vi "Module Execution Main.vi"() -> ()   [LabVIEW 2013, in "module execution process.lvlib"]
uses:
  module execution process.lvlib
  SubVIs/queue name.ctl
  SubVIs/command commands to rtexe process.ctl
  <vilib>/NI/Module Execution Interface/Engine Runtime/Engine Runtime Interface.lvclass
  <vilib>/NI/Tag Bus Module Framework/plugin discovery singleton/class discovery singleton methods.ctl
  SubVIs/engine status data.ctl
  <vilib>/NI/Module Execution Interface/Engine Runtime/Execution States.ctl
  <vilib>/NI/AMC/Read Termination Message.vi
  <vilib>/NI/AMC/Create Single Message.vi
  <vilib>/NI/AMC/Globals.vi
  <vilib>/NI/Module Execution Interface/Engine Configuration/engine configuration.lvclass
  <vilib>/NI/Tag Bus Module Framework/module configuration/TBM module configuration.lvclass
  <vilib>/NI/Tag Bus Module Framework/runtime/TBM module execution interface.lvclass
  <vilib>/nisyscfg/nisyscfg.lvlib
  Framework Configuration Classes/platypus configuration/PLConfigurationSerializer.lvlib
  <vilib>/NI/Tag Bus Module Framework/plugin discovery singleton/class discovery singleton.lvlib
  <vilib>/NI/AMC/AMC.lvlib
panel:
  out "error out":errorcluster
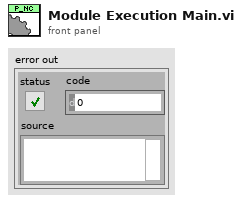
[diagram p1: front panel]
types:
  T1 = typedef "module execution process.lvlib/command commands to rtexe process.ctl" = enum16{"Initialize", "Load from File", "Load from String", "Open All Engines", "Open Single Engine", "Initialize All Engines", "Initialize Single Engine", "Start All", "Start Single", "Pause All", "Pause Single", "Stop All", "Stop Single", "Close All", "Close Single", "Set Safe State All", "Set Safe State Single", "Get Status", "Exit", "Error", "Add Search Paths"}
  T2 = typedef "module execution process.lvlib/queue name.ctl" = enum16{"TOrtmainexec", "FROMrtmainexec"}
  T3 = typedef "AMC.lvlib/Message Queue.ctl" = refnum<queue>
  T4 = typedef "class discovery singleton.lvlib/class discovery singleton methods.ctl" = enum16{"add search paths", "load class by name", "list available classes", "get class path"}
  T5 = typedef "module execution process.lvlib/engine status data.ctl" = cluster{"Name":string, "Engine State":T6, "Engine Error":errorcluster}
  T6 = typedef "Engine Runtime Interface.lvclass/Execution States.ctl" = enum16{"Initializing", "Paused (Initialized)", "Running", "Set Safe Outputs", "Uninitializing", "Stopped (Uninitialized)", "Error (Uninitialized)", "Safe State (Uninitialized)", "Closed"}
  T7 = typedef "module execution process.lvlib/configuration elements.ctl" = cluster{"Name":string, "opened?":bool, "configuration":T8, "engine":refnum<class "Engine Runtime Interface.lvclass">, "modules":refnum<class "TBM module execution interface.lvclass">[]}
  T8 = typedef "PLConfigurationSerializer.lvlib/engines cluster.ctl" = cluster{"engine configuration":refnum<class "engine configuration.lvclass">, "modules":refnum<class "TBM module configuration.lvclass">[]}
  T9 = typedef "PLConfigurationSerializer.lvlib/systems cluster.ctl" = cluster{"System Configuration":refnum<class "PL_System Configuration.lvclass">, "targets":T10[]}
  T10 = typedef "PLConfigurationSerializer.lvlib/targets cluster.ctl" = cluster{"Target Configuration":refnum<class "PL_Target Configuration.lvclass">, "engines":T8[]}
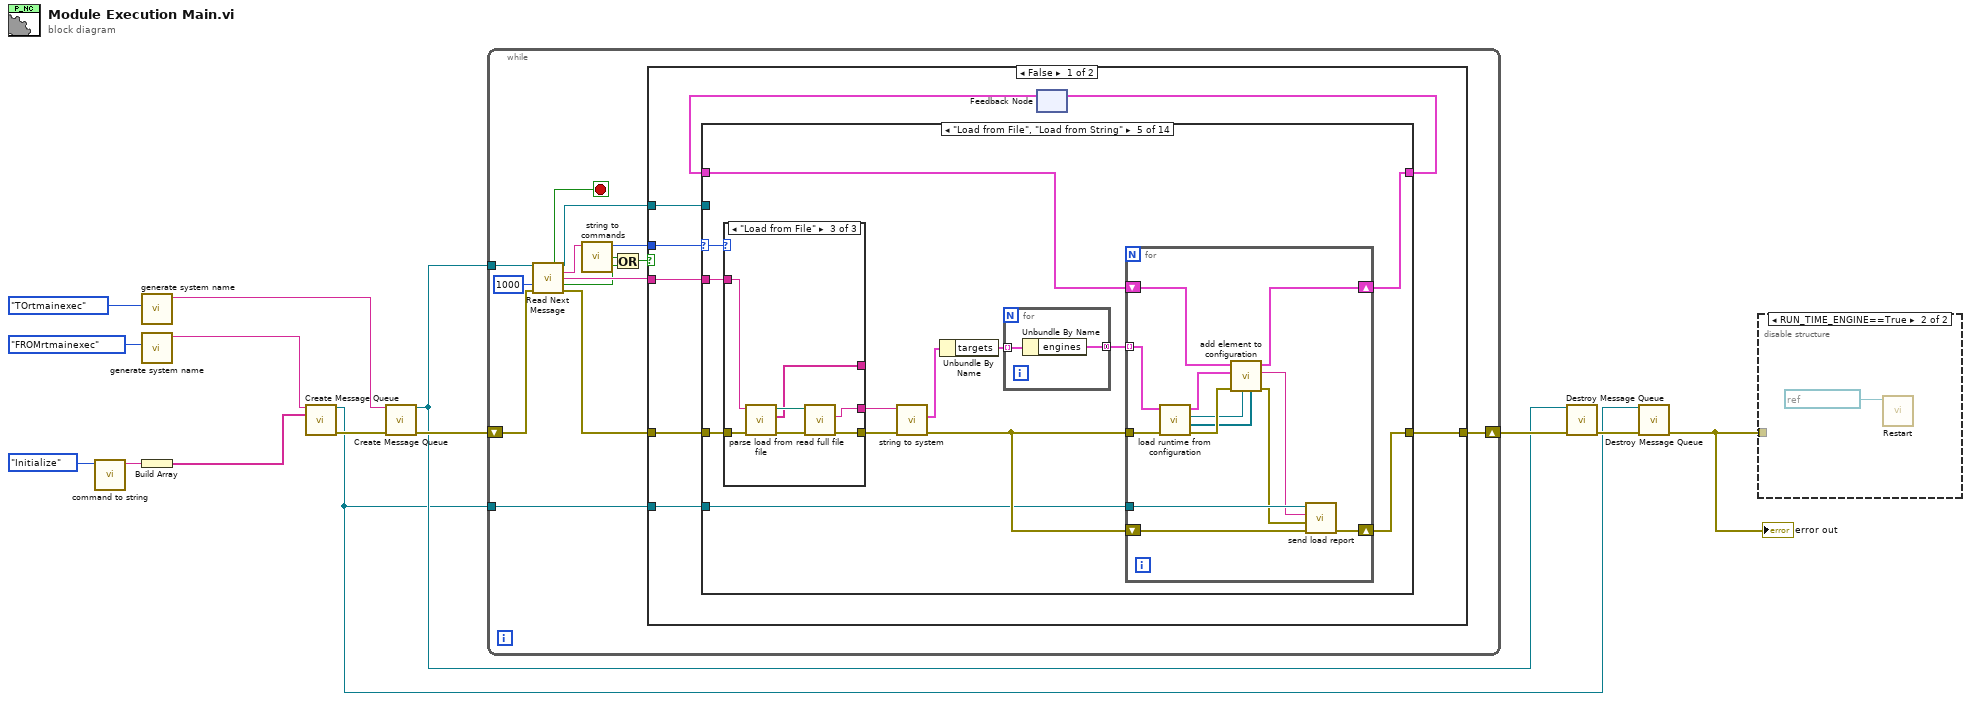
[diagram p0: block diagram]
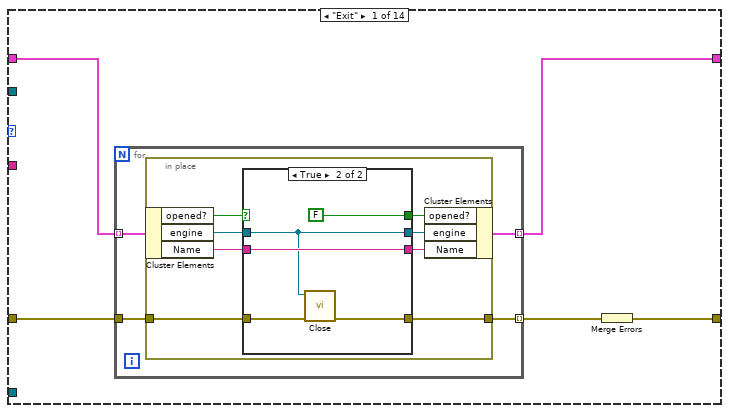
[diagram p3: hidden frame]
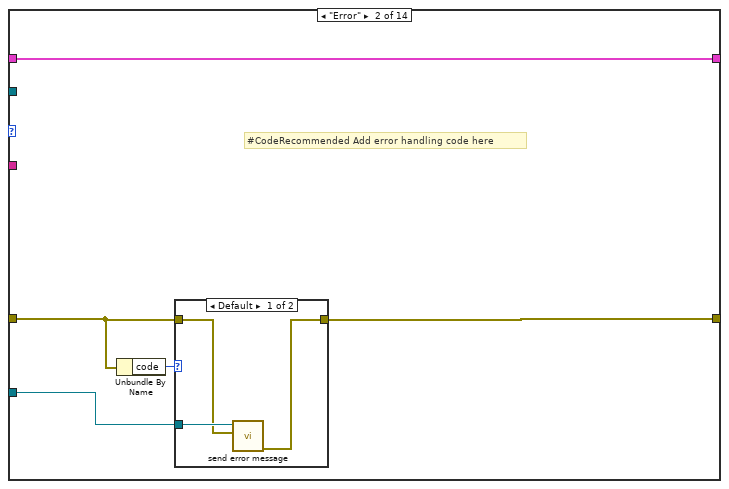
[diagram p5: hidden frame]
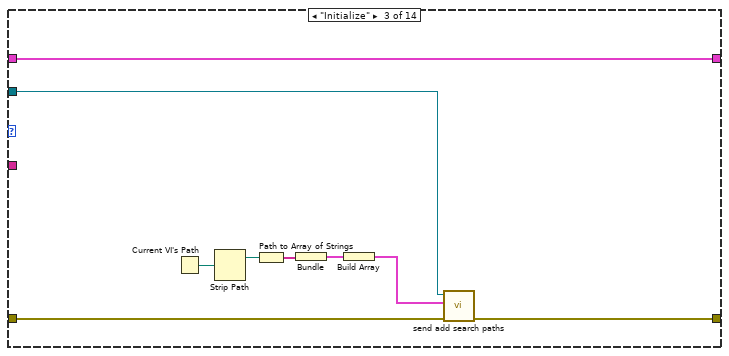
[diagram p7: hidden frame]
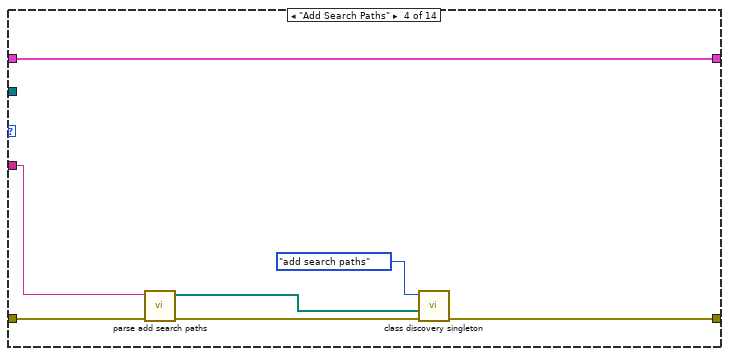
[diagram p8: hidden frame]
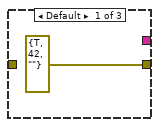
[diagram p9: hidden frame]
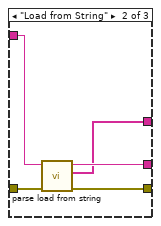
[diagram p10: hidden frame]
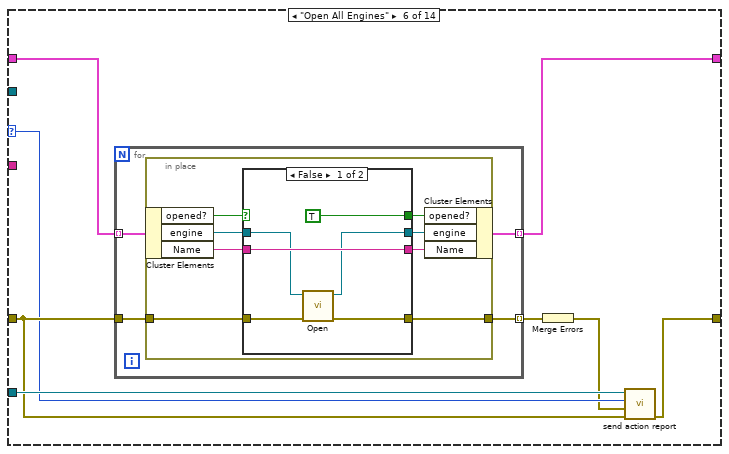
[diagram p11: hidden frame]
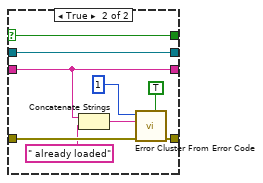
[diagram p12: hidden frame]
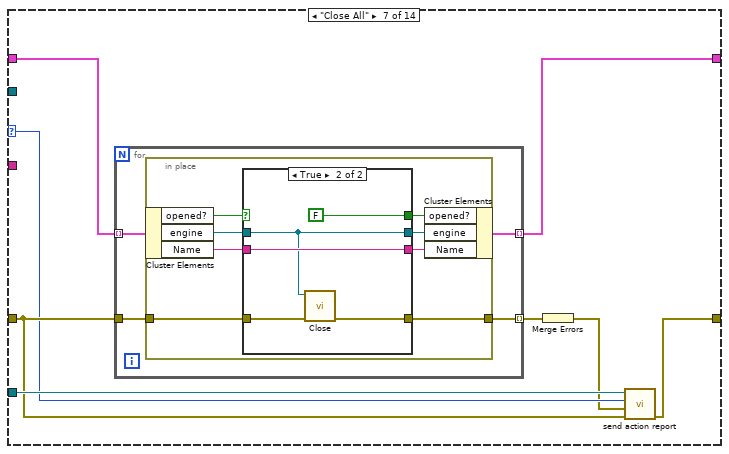
[diagram p13: hidden frame]
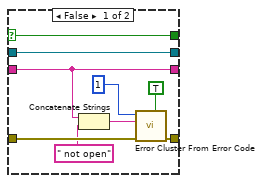
[diagram p14: hidden frame]
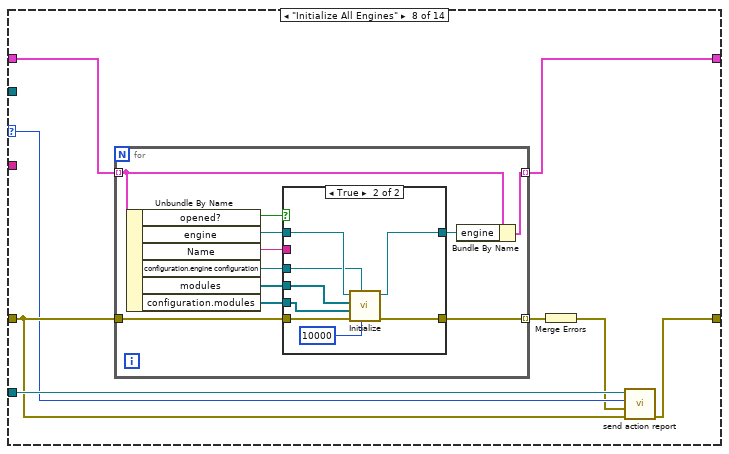
[diagram p15: hidden frame]
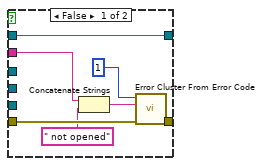
[diagram p16: hidden frame]
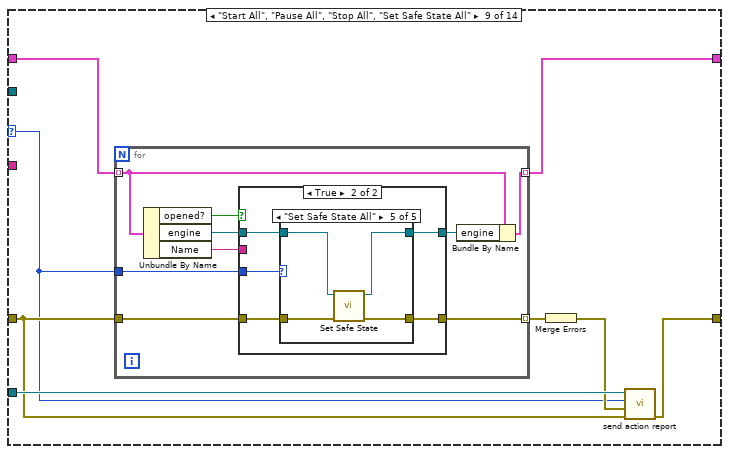
[diagram p17: hidden frame]
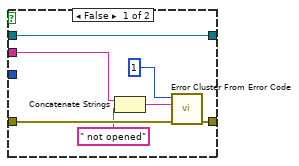
[diagram p18: hidden frame]
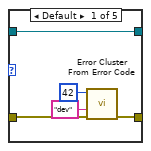
[diagram p19: hidden frame]
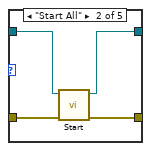
[diagram p20: hidden frame]
diagram:
  n1 = call "command to string.vi"("commands"=command_commands_to_rtexe_process."Initialize") -> ("command string"=w6:string)  [unwired: 10 in]
  n2 = call "generate system name.vi"("queue"=queue_name."TOrtmainexec") -> ("queue name"=w11:string)  [unwired: 10 in]
  n3 = call "generate system name.vi"("queue"=queue_name."FROMrtmainexec") -> ("queue name"=w13:string)  [unwired: 10 in]
  n4 = Build Array(w6) -> (w5:string[])
  n5 = call <vilib>:"Create Message Queue.vi"("message queue name"=w13, "initial message names"=w5) -> ("message queue out"=w1:T3, "error out"=w12:errorcluster)  [unwired: 12 in]
  n6 = call <vilib>:"Create Message Queue.vi"("message queue name"=w11, "error in"=w12) -> ("message queue out"=w2:T3, "error out"=w10:errorcluster)  [unwired: 12 in]
  n7 = while {
    tunnel: w2 -> [w26]
    shift-right: [w28] -> w14
    shift-left: w10 -> [w23]
    tunnel: w1 -> [w27]
    stop <- w25 stop-if-true
    n8 = call <vilib>:"Read Next Message.vi"("message queue in"=w26, "timeout (1 ms)"=1000, "error in"=w23) -> ("exit process?"=w25:bool, "message queue out"=w15:T3, "message name"=w20:string, "message value"=w24:string, "timed out?"=w18:bool, "error out"=w22:errorcluster)  [unwired: 5 in, 2 out]
    n9 = call "string to commands.vi"("command string"=w20) -> ("invalid"=w19:bool, "commands"=w16:T1)  [unwired: 9 in]
    n10 = Or(x=w19, y=w18) -> (x .or. y?=w17:bool)
    n11 = case shown="False" w17 {
      tunnel: w24 -> [w36 _]
      tunnel: [w35 w546] -> w28
      tunnel: w27 -> [w34 _]
      tunnel: w22 -> [w33 w546]
      tunnel: w16 -> [w32 _]
      tunnel: w15 -> [w31 _]
      frame False {
        n12 = feedback #1() -> (w29:T7[])  [unwired: 1 in]
        n13 = case shown="\"Load from File\", \"Load from String\"" w32 {
          selector: w32 -> [_ _ _ _ w97 w129 w164 w198 w231 w290 w348 w405 w450 _]
          tunnel: w36 -> [_ _ _ w80 w99 _ _ _ _ w287 w345 w402 w457 _]
          tunnel: [w40 w67 w79 w86 w91 w134 w169 w203 w237 w293 w351 w408 w462 w522] -> w30
          tunnel: w29 -> [w41 w67 w79 w86 w90 w135 w170 w204 w238 w294 w352 w409 w463 w523]
          tunnel: [w37 w64 w77 w84 w88 w131 w166 w200 w234 w291 w349 w406 w460 w520] -> w35
          tunnel: w33 -> [w39 w65 w78 w83 w98 w132 w167 w201 w235 w289 w347 w404 w459 w521]
          tunnel: w34 -> [_ w63 _ _ w87 w133 w168 w202 w236 w292 w350 w407 w461 w519]
          tunnel: w31 -> [_ _ w76 _ _ _ _ _ _ _ _ _ _ _]
          frame "Exit" {
            n14 = for {
              tunnel: w41 -> [w45] mode=indexing
              tunnel: [w44] -> w40 mode=indexing
              tunnel: w39 -> [w43]
              tunnel: [w42] -> w38 mode=indexing
              n15 = in-place {
                in-place-border: w43 -> [w50]
                in-place-border: [w49] -> w42
                n16 = in-place-cluster #2(w45) -> ("opened?"=w53:bool, "engine"=w52:refnum<class "Engine Runtime Interface.lvclass">, "Name"=w48:string)
                n17 = case shown="True" w53 {
                  selector: w53 -> [w54 _]
                  tunnel: w52 -> [w57 w58]
                  tunnel: [w57 w58] -> w51
                  tunnel: w50 -> [w56 w60]
                  tunnel: [w56 w59] -> w49
                  tunnel: w48 -> [w55 w62]
                  tunnel: [w55 w62] -> w47
                  tunnel: [w54 FALSE ("opened?")] -> w46
                  frame False {
                  }
                  frame True {
                    n18 = call-dynamic "Close.vi"("error in"=w60, "Engine Runtime Interface in"=w58) -> ("error out"=w59:errorcluster)  [unwired: 9 in]
                  }
                }
                n19 = in-place-cluster #2("opened?"=w46, "engine"=w51, "Name"=w47) -> (w44:T7)
              }
            }
            n20 = Merge Errors(w38) -> (w37:errorcluster)
          }
          frame "Error" {
            # "#CodeRecommended Add error handling code here"
            n21 = Unbundle By Name(w65) -> ("code"=w66:i32)
            n22 = case shown="Default" w66 {
              tunnel: w65 -> [w68 _]
              tunnel: [w69 _] -> w64
              tunnel: w63 -> [w70 _]
              frame Default {
                n23 = call "send error message.vi"("error to send"=w68, "message queue in"=w70) -> ("error out"=w69:errorcluster)  [unwired: 8 in, 1 out]
              }
              frame 538255 {
                # "Ignore this timeout error for now."
              }
            }
          }
          frame "Initialize" {
            n24 = Current VI's Path() -> (path=w75:path)
            n25 = Strip Path(path=w75) -> (stripped path=w74:path)  [unwired: 1 out]
            n26 = Path to Array of Strings(0:w74) -> (2:w73:string[])  [unwired: 1 out]
            n27 = Bundle("array of strings"=w73) -> (w72:cluster{"array of strings":string[]})  [unwired: 1 in]
            n28 = Build Array(w72) -> (w71:cluster{"array of strings":string[]}[])
            n29 = call "send add search paths.vi"("error in"=w78, "search paths"=w71, "message queue in"=w76) -> ("error out"=w77:errorcluster)  [unwired: 7 in, 1 out]
          }
          frame "Add Search Paths" {
            n30 = call "parse add search paths.vi"("error in"=w83, "message data"=w80) -> ("error out"=w82:errorcluster, "paths"=w81:path[])  [unwired: 8 in]
            n31 = call <vilib>:"class discovery singleton.vi"("error in"=w82, "Plugin Search Paths"=w81, "method"=class_discovery_singleton_methods."add search paths") -> ("error out"=w84:errorcluster)  [unwired: 5 in, 3 out]
          }
          frame "Load from File", "Load from String" {
            n32 = case shown="\"Load from File\"" w97 {
              tunnel: w99 -> [_ w118 w126]
              tunnel: w98 -> [_ w120 w127]
              tunnel: [errorcluster {"status"=TRUE, "code"=42, "source"=""} ("error out") w119 w121] -> w96
              tunnel: [_ w116 w123] -> _
              tunnel: [_ w117 w122] -> w95
              frame Default {
              }
              frame "Load from String" {
                n33 = call "parse load from string.vi"("error in"=w120, "message data"=w118) -> ("error out"=w119:errorcluster, "targets to load"=w116:string[], "system data"=w117:string)  [unwired: 7 in]
              }
              frame "Load from File" {
                n34 = call "parse load from file.vi"("error in"=w127, "message data"=w126) -> ("error out"=w125:errorcluster, "targets to load"=w123:string[], "path"=w124:path)  [unwired: 7 in]
                n35 = call "read full file.vi"("error in"=w125, "file path"=w124) -> ("error out"=w121:errorcluster, "data"=w122:string)  [unwired: 8 in]
              }
            }
            n36 = call "string to system.vi"("error in"=w96, "data"=w95) -> ("error out"=w89:errorcluster, "system"=w94:T9)  [unwired: 8 in]
            n37 = Unbundle By Name(w94) -> ("targets"=w93:T10[])
            n38 = for {
              tunnel: w93 -> [w114] mode=indexing
              tunnel: [w113] -> w92 mode=concatenating
              n39 = Unbundle By Name(w114) -> ("engines"=w113:T8[])
            }
            n40 = for {
              tunnel: w92 -> [w111] mode=indexing
              tunnel: w89 -> [w112]
              shift-right: [w106] -> w91
              shift-left: w90 -> [w105]
              shift-right: [w102] -> w88
              shift-left: w89 -> [w103]
              tunnel: w87 -> [w104]
              n41 = call "load runtime from configuration.vi"("error in"=w112, "engine configuration in"=w111) -> ("error out"=w110:errorcluster, "Component Runtime Objects"=w107:refnum<class "TBM module execution interface.lvclass">[], "Engine Runtime Object"=w108:refnum<class "Engine Runtime Interface.lvclass">, "engine configuration out"=w109:T8)  [unwired: 6 in]
              n42 = call "add element to configuration.vi"("Component Runtime Objects"=w107, "Engine Runtime Object"=w108, "error in"=w110, "engine configuration out"=w109, "Configuration in"=w105) -> ("error out"=w100:errorcluster, "engine loaded"=w101:string, "Configuration out"=w106:T7[])  [unwired: 4 in]
              n43 = call "send load report.vi"("error in"=w103, "load error"=w100, "engine loaded"=w101, "message queue in"=w104) -> ("error out"=w102:errorcluster)  [unwired: 6 in, 1 out]
            }
          }
          frame "Open All Engines" {
            n44 = for {
              tunnel: w135 -> [w139] mode=indexing
              tunnel: [w138] -> w134 mode=indexing
              tunnel: w132 -> [w137]
              tunnel: [w136] -> w130 mode=indexing
              n45 = in-place {
                in-place-border: w137 -> [w144]
                in-place-border: [w143] -> w136
                n46 = in-place-cluster #3(w139) -> ("opened?"=w147:bool, "engine"=w146:refnum<class "Engine Runtime Interface.lvclass">, "Name"=w142:string)
                n47 = case shown="False" w147 {
                  selector: w147 -> [_ w154]
                  tunnel: w146 -> [w150 w162]
                  tunnel: [w149 w162] -> w145
                  tunnel: w144 -> [w153 w161]
                  tunnel: [w152 w160] -> w143
                  tunnel: w142 -> [w151 w155]
                  tunnel: [w151 w155] -> w141
                  tunnel: [TRUE ("opened?") w154] -> w140
                  frame False {
                    n48 = call-dynamic "Open.vi"("error in"=w153, "Engine Runtime Interface in"=w150) -> ("error out"=w152:errorcluster, "Engine Runtime Interface out"=w149:refnum<class "Engine Runtime Interface.lvclass">)  [unwired: 8 in]
                  }
                  frame True {
                    n49 = Concatenate Strings(w155, " already loaded" ("string")) -> (w157:string)
                    n50 = call <vilib>:"Error Cluster From Error Code.vi"("is warning? (False)"=TRUE, "error in (no error)"=w161, "error message (\"\")"=w157, "error code (0)"=1) -> ("error out"=w160:errorcluster)  [unwired: 5 in]
                  }
                }
                n51 = in-place-cluster #3("opened?"=w140, "engine"=w145, "Name"=w141) -> (w138:T7)
              }
            }
            n52 = Merge Errors(w130) -> (w128:errorcluster)
            n53 = call "send action report.vi"("error in"=w132, "command error"=w128, "commands"=w129, "message queue in"=w133) -> ("error out"=w131:errorcluster)  [unwired: 6 in, 1 out]
          }
          frame "Close All" {
            n54 = for {
              tunnel: w170 -> [w174] mode=indexing
              tunnel: [w173] -> w169 mode=indexing
              tunnel: w167 -> [w172]
              tunnel: [w171] -> w165 mode=indexing
              n55 = in-place {
                in-place-border: w172 -> [w179]
                in-place-border: [w178] -> w171
                n56 = in-place-cluster #4(w174) -> ("opened?"=w182:bool, "engine"=w181:refnum<class "Engine Runtime Interface.lvclass">, "Name"=w177:string)
                n57 = case shown="True" w182 {
                  selector: w182 -> [w183 _]
                  tunnel: w181 -> [w191 w192]
                  tunnel: [w191 w192] -> w180
                  tunnel: w179 -> [w190 w194]
                  tunnel: [w189 w193] -> w178
                  tunnel: w177 -> [w184 w196]
                  tunnel: [w184 w196] -> w176
                  tunnel: [w183 FALSE ("opened?")] -> w175
                  frame False {
                    n58 = Concatenate Strings(w184, " not open" ("string")) -> (w186:string)
                    n59 = call <vilib>:"Error Cluster From Error Code.vi"("is warning? (False)"=TRUE, "error in (no error)"=w190, "error message (\"\")"=w186, "error code (0)"=1) -> ("error out"=w189:errorcluster)  [unwired: 5 in]
                  }
                  frame True {
                    n60 = call-dynamic "Close.vi"("error in"=w194, "Engine Runtime Interface in"=w192) -> ("error out"=w193:errorcluster)  [unwired: 9 in]
                  }
                }
                n61 = in-place-cluster #4("opened?"=w175, "engine"=w180, "Name"=w176) -> (w173:T7)
              }
            }
            n62 = Merge Errors(w165) -> (w163:errorcluster)
            n63 = call "send action report.vi"("error in"=w167, "command error"=w163, "commands"=w164, "message queue in"=w168) -> ("error out"=w166:errorcluster)  [unwired: 6 in, 1 out]
          }
          frame "Initialize All Engines" {
            n64 = for {
              tunnel: w204 -> [w215] mode=indexing
              tunnel: [w214] -> w203 mode=indexing
              tunnel: w201 -> [w213]
              tunnel: [w212] -> w199 mode=indexing
              n65 = Unbundle By Name(w215) -> ("opened?"=w211:bool, "engine"=w210:refnum<class "Engine Runtime Interface.lvclass">, "Name"=w208:string, "configuration.engine configuration"=w207:refnum<class "engine configuration.lvclass">, "modules"=w206:refnum<class "TBM module execution interface.lvclass">[], "configuration.modules"=w205:refnum<class "TBM module configuration.lvclass">[])
              n66 = case shown="True" w211 {
                tunnel: w210 -> [w222 w227]
                tunnel: [w222 w228] -> w209
                tunnel: w213 -> [w221 w229]
                tunnel: [w220 w230] -> w212
                tunnel: w208 -> [w216 _]
                tunnel: w207 -> [_ w226]
                tunnel: w206 -> [_ w225]
                tunnel: w205 -> [_ w224]
                frame False {
                  n67 = Concatenate Strings(w216, " not opened" ("string")) -> (w218:string)
                  n68 = call <vilib>:"Error Cluster From Error Code.vi"("error in (no error)"=w221, "error message (\"\")"=w218, "error code (0)"=1) -> ("error out"=w220:errorcluster)  [unwired: 6 in]
                }
                frame True {
                  n69 = call-dynamic "Initialize.vi"("timeout in ms"=10000, "Engine Configuration"=w226, "error in"=w229, "module Configurations"=w224, "modules"=w225, "Engine Runtime Interface in"=w227) -> ("error out"=w230:errorcluster, "Engine Runtime Interface out"=w228:refnum<class "Engine Runtime Interface.lvclass">)  [unwired: 4 in]
                }
              }
              n70 = Bundle By Name(cluster=w215, "engine"=w209) -> (w214:T7)
            }
            n71 = Merge Errors(w199) -> (w197:errorcluster)
            n72 = call "send action report.vi"("error in"=w201, "command error"=w197, "commands"=w198, "message queue in"=w202) -> ("error out"=w200:errorcluster)  [unwired: 6 in, 1 out]
          }
          frame "Start All", "Pause All", "Stop All", "Set Safe State All" {
            n73 = for {
              tunnel: w238 -> [w247] mode=indexing
              tunnel: [w246] -> w237 mode=indexing
              tunnel: w235 -> [w245]
              tunnel: [w244] -> w233 mode=indexing
              tunnel: w231 -> [w239]
              n74 = Unbundle By Name(w247) -> ("opened?"=w243:bool, "engine"=w242:refnum<class "Engine Runtime Interface.lvclass">, "Name"=w240:string)
              n75 = case shown="True" w243 {
                tunnel: w242 -> [w254 w256]
                tunnel: [w254 w257] -> w241
                tunnel: w245 -> [w253 w259]
                tunnel: [w252 w258] -> w244
                tunnel: w240 -> [w248 _]
                tunnel: w239 -> [_ w255]
                frame False {
                  n76 = Concatenate Strings(w248, " not opened" ("string")) -> (w250:string)
                  n77 = call <vilib>:"Error Cluster From Error Code.vi"("error in (no error)"=w253, "error message (\"\")"=w250, "error code (0)"=1) -> ("error out"=w252:errorcluster)  [unwired: 6 in]
                }
                frame True {
                  n78 = case shown="\"Set Safe State All\"" w255 {
                    tunnel: w259 -> [w262 w268 w272 w276 w280]
                    tunnel: [w263 w267 w271 w275 w279] -> w258
                    tunnel: [w264 w266 w270 w273 w278] -> w257
                    tunnel: w256 -> [w264 w265 w269 w274 w277]
                    frame Default {
                      n79 = call <vilib>:"Error Cluster From Error Code.vi"("error in (no error)"=w262, "error message (\"\")"="dev" ("error message (\"\")"), "error code (0)"=42) -> ("error out"=w263:errorcluster)  [unwired: 6 in]
                    }
                    frame "Start All" {
                      n80 = call-dynamic "Start.vi"("error in"=w268, "Engine Runtime Interface in"=w265) -> ("error out"=w267:errorcluster, "Engine Runtime Interface out"=w266:refnum<class "Engine Runtime Interface.lvclass">)  [unwired: 8 in]
                    }
                    frame "Pause All" {
                      n81 = call-dynamic "Pause.vi"("error in"=w272, "Engine Runtime Interface in"=w269) -> ("error out"=w271:errorcluster, "Engine Runtime Interface out"=w270:refnum<class "Engine Runtime Interface.lvclass">)  [unwired: 8 in]
                    }
                    frame "Stop All" {
                      n82 = call-dynamic "Stop.vi"("error in"=w276, "Engine Runtime Interface in"=w274) -> ("error out"=w275:errorcluster, "Engine Runtime Interface out"=w273:refnum<class "Engine Runtime Interface.lvclass">)  [unwired: 8 in]
                    }
                    frame "Set Safe State All" {
                      n83 = call-dynamic "Set Safe State.vi"("error in"=w280, "Engine Runtime Interface in"=w277) -> ("error out"=w279:errorcluster, "Engine Runtime Interface out"=w278:refnum<class "Engine Runtime Interface.lvclass">)  [unwired: 8 in]
                    }
                  }
                }
              }
              n84 = Bundle By Name(cluster=w247, "engine"=w241) -> (w246:T7)
            }
            n85 = Merge Errors(w233) -> (w232:errorcluster)
            n86 = call "send action report.vi"("error in"=w235, "command error"=w232, "commands"=w231, "message queue in"=w236) -> ("error out"=w234:errorcluster)  [unwired: 6 in, 1 out]
          }
          frame "Open Single Engine" {
            n87 = call "parse single action command.vi"("error in"=w289, "message data"=w287) -> ("error out"=w288:errorcluster, "engine name"=w286:string)  [unwired: 8 in]
            n88 = for {
              tunnel: w294 -> [w301] mode=indexing
              tunnel: [w300] -> w293 mode=indexing
              tunnel: w286 -> [w297]
              tunnel: [w296] -> w285 mode=indexing
              tunnel: w288 -> [w299]
              tunnel: [w298] -> w283
              stop <- w295 stop-if-true
              n89 = in-place {
                in-place-border: w299 -> [w308]
                in-place-border: [w307] -> w298
                in-place-border: w297 -> [w304]
                in-place-border: [w302] -> w296
                in-place-border: [w302] -> w295
                n90 = in-place-cluster #5(w301) -> ("opened?"=w311:bool, "engine"=w310:refnum<class "Engine Runtime Interface.lvclass">, "Name"=w303:string)
                n91 = Equal?(x=w303, y=w304) -> (x = y?=w302:bool)
                n92 = case shown="True" w302 {
                  tunnel: w311 -> [w315 w323]
                  tunnel: w310 -> [w314 w322]
                  tunnel: [w314 w321] -> w309
                  tunnel: w308 -> [w312 w320]
                  tunnel: [w312 w319] -> w307
                  tunnel: [w313 w318] -> w306
                  tunnel: [w315 w317] -> w305
                  tunnel: w303 -> [w313 w316]
                  frame False {
                  }
                  frame True {
                    n93 = case shown="False" w323 {
                      selector: w323 -> [_ w330]
                      tunnel: w322 -> [w326 w338]
                      tunnel: [w325 w338] -> w321
                      tunnel: w320 -> [w329 w337]
                      tunnel: [w328 w336] -> w319
                      tunnel: w316 -> [w327 w331]
                      tunnel: [w327 w331] -> w318
                      tunnel: [TRUE ("opened?") w330] -> w317
                      frame False {
                        n94 = call-dynamic "Open.vi"("error in"=w329, "Engine Runtime Interface in"=w326) -> ("error out"=w328:errorcluster, "Engine Runtime Interface out"=w325:refnum<class "Engine Runtime Interface.lvclass">)  [unwired: 8 in]
                      }
                      frame True {
                        n95 = Concatenate Strings(w331, " already loaded" ("string")) -> (w333:string)
                        n96 = call <vilib>:"Error Cluster From Error Code.vi"("is warning? (False)"=TRUE, "error in (no error)"=w337, "error message (\"\")"=w333, "error code (0)"=1) -> ("error out"=w336:errorcluster)  [unwired: 5 in]
                      }
                    }
                  }
                }
                n97 = in-place-cluster #5("opened?"=w305, "engine"=w309, "Name"=w306) -> (w300:T7)
              }
            }
            n98 = Or Array Elements(Boolean array=w285) -> (logical OR=w284:bool)
            n99 = Select(t=w283, s=w284, f=errorcluster {"status"=TRUE, "code"=1, "source"="Not found"}) -> (s? t:f=w282:errorcluster)
            n100 = call "send action report.vi"("error in"=w288, "command error"=w282, "commands"=w290, "message queue in"=w292) -> ("error out"=w291:errorcluster)  [unwired: 6 in, 1 out]
          }
          frame "Close Single" {
            n101 = call "parse single action command.vi"("error in"=w347, "message data"=w345) -> ("error out"=w346:errorcluster, "engine name"=w344:string)  [unwired: 8 in]
            n102 = for {
              tunnel: w352 -> [w359] mode=indexing
              tunnel: [w358] -> w351 mode=indexing
              tunnel: w344 -> [w355]
              tunnel: [w354] -> w343 mode=indexing
              tunnel: w346 -> [w357]
              tunnel: [w356] -> w341
              stop <- w353 stop-if-true
              n103 = in-place {
                in-place-border: w357 -> [w366]
                in-place-border: [w365] -> w356
                in-place-border: w355 -> [w362]
                in-place-border: [w360] -> w354
                in-place-border: [w360] -> w353
                n104 = in-place-cluster #6(w359) -> ("opened?"=w369:bool, "engine"=w368:refnum<class "Engine Runtime Interface.lvclass">, "Name"=w361:string)
                n105 = Equal?(x=w361, y=w362) -> (x = y?=w360:bool)
                n106 = case shown="True" w360 {
                  tunnel: w369 -> [w373 w381]
                  tunnel: w368 -> [w372 w380]
                  tunnel: [w372 w379] -> w367
                  tunnel: w366 -> [w370 w378]
                  tunnel: [w370 w377] -> w365
                  tunnel: [w371 w376] -> w364
                  tunnel: [w373 w375] -> w363
                  tunnel: w361 -> [w371 w374]
                  frame False {
                  }
                  frame True {
                    n107 = case shown="True" w381 {
                      selector: w381 -> [w382 _]
                      tunnel: w380 -> [w390 w391]
                      tunnel: [w390 w391] -> w379
                      tunnel: w378 -> [w389 w392]
                      tunnel: [w388 w393] -> w377
                      tunnel: w374 -> [w383 w395]
                      tunnel: [w383 w395] -> w376
                      tunnel: [w382 FALSE ("opened?")] -> w375
                      frame False {
                        n108 = Concatenate Strings(w383, " not opened" ("string")) -> (w385:string)
                        n109 = call <vilib>:"Error Cluster From Error Code.vi"("is warning? (False)"=TRUE, "error in (no error)"=w389, "error message (\"\")"=w385, "error code (0)"=1) -> ("error out"=w388:errorcluster)  [unwired: 5 in]
                      }
                      frame True {
                        n110 = call-dynamic "Close.vi"("error in"=w392, "Engine Runtime Interface in"=w391) -> ("error out"=w393:errorcluster)  [unwired: 9 in]
                      }
                    }
                  }
                }
                n111 = in-place-cluster #6("opened?"=w363, "engine"=w367, "Name"=w364) -> (w358:T7)
              }
            }
            n112 = Or Array Elements(Boolean array=w343) -> (logical OR=w342:bool)
            n113 = Select(t=w341, s=w342, f=errorcluster {"status"=TRUE, "code"=1, "source"="Not found"}) -> (s? t:f=w340:errorcluster)
            n114 = call "send action report.vi"("error in"=w346, "command error"=w340, "commands"=w348, "message queue in"=w350) -> ("error out"=w349:errorcluster)  [unwired: 6 in, 1 out]
          }
          frame "Initialize Single Engine" {
            n115 = call "parse single action command.vi"("error in"=w404, "message data"=w402) -> ("error out"=w403:errorcluster, "engine name"=w401:string)  [unwired: 8 in]
            n116 = for {
              tunnel: w409 -> [w422] mode=indexing
              tunnel: [w421] -> w408 mode=indexing
              tunnel: w401 -> [w418]
              tunnel: [w417] -> w400 mode=indexing
              tunnel: w403 -> [w420]
              tunnel: [w419] -> w398
              stop <- w417 stop-if-true
              n117 = Unbundle By Name(w422) -> ("configuration.engine configuration"=w410:refnum<class "engine configuration.lvclass">, "opened?"=w416:bool, "engine"=w415:refnum<class "Engine Runtime Interface.lvclass">, "modules"=w411:refnum<class "TBM module execution interface.lvclass">[], "configuration.modules"=w412:refnum<class "TBM module configuration.lvclass">[], "Name"=w413:string)
              n118 = Equal?(x=w413, y=w418) -> (x = y?=w417:bool)
              n119 = case shown="True" w417 {
                tunnel: w416 -> [_ w433]
                tunnel: w415 -> [w424 w432]
                tunnel: [w424 w431] -> w414
                tunnel: w420 -> [w423 w430]
                tunnel: [w423 w429] -> w419
                tunnel: w413 -> [_ w428]
                tunnel: w412 -> [_ w427]
                tunnel: w411 -> [_ w426]
                tunnel: w410 -> [_ w425]
                frame False {
                }
                frame True {
                  n120 = case shown="True" w433 {
                    tunnel: w432 -> [w441 w447]
                    tunnel: [w441 w446] -> w431
                    tunnel: w430 -> [w440 w448]
                    tunnel: [w439 w445] -> w429
                    tunnel: w428 -> [w434 _]
                    tunnel: w427 -> [_ w444]
                    tunnel: w426 -> [_ w443]
                    tunnel: w425 -> [_ w442]
                    frame False {
                      n121 = Concatenate Strings(w434, " not opened" ("string")) -> (w436:string)
                      n122 = call <vilib>:"Error Cluster From Error Code.vi"("is warning? (False)"=TRUE, "error in (no error)"=w440, "error message (\"\")"=w436, "error code (0)"=1) -> ("error out"=w439:errorcluster)  [unwired: 5 in]
                    }
                    frame True {
                      n123 = call-dynamic "Initialize.vi"("timeout in ms"=10000, "Engine Configuration"=w442, "error in"=w448, "module Configurations"=w444, "modules"=w443, "Engine Runtime Interface in"=w447) -> ("error out"=w445:errorcluster, "Engine Runtime Interface out"=w446:refnum<class "Engine Runtime Interface.lvclass">)  [unwired: 4 in]
                    }
                  }
                }
              }
              n124 = Bundle By Name(cluster=w422, "engine"=w414) -> (w421:T7)
            }
            n125 = Or Array Elements(Boolean array=w400) -> (logical OR=w399:bool)
            n126 = Select(t=w398, s=w399, f=errorcluster {"status"=TRUE, "code"=1, "source"="Not found"}) -> (s? t:f=w397:errorcluster)
            n127 = call "send action report.vi"("error in"=w403, "command error"=w397, "commands"=w405, "message queue in"=w407) -> ("error out"=w406:errorcluster)  [unwired: 6 in, 1 out]
          }
          frame "Start Single", "Pause Single", "Stop Single", "Set Safe State Single" {
            n128 = call "parse single action command.vi"("error in"=w459, "message data"=w457) -> ("error out"=w458:errorcluster, "engine name"=w456:string)  [unwired: 8 in]
            n129 = for {
              tunnel: w463 -> [w474] mode=indexing
              tunnel: [w473] -> w462 mode=indexing
              tunnel: w456 -> [w470]
              tunnel: [w469] -> w455 mode=indexing
              tunnel: w458 -> [w472]
              tunnel: [w471] -> w453
              tunnel: w450 -> [w464]
              stop <- w469 stop-if-true
              n130 = Unbundle By Name(w474) -> ("opened?"=w468:bool, "engine"=w467:refnum<class "Engine Runtime Interface.lvclass">, "Name"=w465:string)
              n131 = Equal?(x=w465, y=w470) -> (x = y?=w469:bool)
              n132 = case shown="True" w469 {
                tunnel: w468 -> [_ w483]
                tunnel: w467 -> [w476 w482]
                tunnel: [w476 w481] -> w466
                tunnel: w472 -> [w475 w480]
                tunnel: [w475 w479] -> w471
                tunnel: w465 -> [_ w478]
                tunnel: w464 -> [_ w477]
                frame False {
                }
                frame True {
                  n133 = case shown="True" w483 {
                    tunnel: w482 -> [w491 w494]
                    tunnel: [w491 w495] -> w481
                    tunnel: w480 -> [w490 w493]
                    tunnel: [w489 w496] -> w479
                    tunnel: w478 -> [w484 _]
                    tunnel: w477 -> [_ w492]
                    frame False {
                      n134 = Concatenate Strings(w484, " not opened" ("string")) -> (w486:string)
                      n135 = call <vilib>:"Error Cluster From Error Code.vi"("is warning? (False)"=TRUE, "error in (no error)"=w490, "error message (\"\")"=w486, "error code (0)"=1) -> ("error out"=w489:errorcluster)  [unwired: 5 in]
                    }
                    frame True {
                      n136 = case shown="\"Set Safe State Single\"" w492 {
                        tunnel: w493 -> [w499 w505 w509 w513 w517]
                        tunnel: [w500 w504 w508 w512 w516] -> w496
                        tunnel: [w501 w503 w507 w511 w514] -> w495
                        tunnel: w494 -> [w501 w502 w506 w510 w515]
                        frame Default {
                          n137 = call <vilib>:"Error Cluster From Error Code.vi"("error in (no error)"=w499, "error message (\"\")"="dev" ("error message (\"\")"), "error code (0)"=42) -> ("error out"=w500:errorcluster)  [unwired: 6 in]
                        }
                        frame "Start Single" {
                          n138 = call-dynamic "Start.vi"("error in"=w505, "Engine Runtime Interface in"=w502) -> ("error out"=w504:errorcluster, "Engine Runtime Interface out"=w503:refnum<class "Engine Runtime Interface.lvclass">)  [unwired: 8 in]
                        }
                        frame "Pause Single" {
                          n139 = call-dynamic "Pause.vi"("error in"=w509, "Engine Runtime Interface in"=w506) -> ("error out"=w508:errorcluster, "Engine Runtime Interface out"=w507:refnum<class "Engine Runtime Interface.lvclass">)  [unwired: 8 in]
                        }
                        frame "Set Safe State Single" {
                          n140 = call-dynamic "Set Safe State.vi"("error in"=w513, "Engine Runtime Interface in"=w510) -> ("error out"=w512:errorcluster, "Engine Runtime Interface out"=w511:refnum<class "Engine Runtime Interface.lvclass">)  [unwired: 8 in]
                        }
                        frame "Stop Single" {
                          n141 = call-dynamic "Stop.vi"("error in"=w517, "Engine Runtime Interface in"=w515) -> ("error out"=w516:errorcluster, "Engine Runtime Interface out"=w514:refnum<class "Engine Runtime Interface.lvclass">)  [unwired: 8 in]
                        }
                      }
                    }
                  }
                }
              }
              n142 = Bundle By Name(cluster=w474, "engine"=w466) -> (w473:T7)
            }
            n143 = Or Array Elements(Boolean array=w455) -> (logical OR=w454:bool)
            n144 = Select(t=w453, s=w454, f=errorcluster {"status"=TRUE, "code"=1, "source"="Not found"}) -> (s? t:f=w452:errorcluster)
            n145 = call "send action report.vi"("error in"=w458, "command error"=w452, "commands"=w450, "message queue in"=w461) -> ("error out"=w460:errorcluster)  [unwired: 6 in, 1 out]
          }
          frame "Get Status" {
            n146 = for {
              tunnel: w523 -> [w534] mode=indexing
              tunnel: [w533] -> w522 mode=indexing
              tunnel: w521 -> [w532]
              tunnel: [w528] -> w518 mode=indexing
              n147 = Unbundle By Name(w534) -> ("Name"=w524:string, "opened?"=w531:bool, "engine"=w530:refnum<class "Engine Runtime Interface.lvclass">)
              n148 = case shown="True" w531 {
                tunnel: w530 -> [w536 w543]
                tunnel: [w536 w540] -> w529
                tunnel: w532 -> [_ w545]
                tunnel: [Execution_States."Closed" ("Engine State") w541] -> w525
                tunnel: [_ w538] -> w526
                frame False {
                }
                frame True {
                  n149 = call-dynamic "Get State.vi"("error in"=w545, "Engine Runtime Interface in"=w543) -> ("error out"=w544:errorcluster, "Engine State"=w541:T6, "Engine Runtime Interface out"=w542:refnum<class "Engine Runtime Interface.lvclass">)  [unwired: 7 in]
                  n150 = call-dynamic "Read Buffered Error.vi"("error in"=w544, "Engine Runtime Interface in"=w542) -> ("error out"=w537:errorcluster, "Engine Error"=w539:errorcluster, "Engine Runtime Interface out"=w540:refnum<class "Engine Runtime Interface.lvclass">)  [unwired: 7 in]
                  n151 = Merge Errors(w539, w537) -> (w538:errorcluster)
                }
              }
              n152 = Bundle By Name(cluster=w534, "engine"=w529) -> (w533:T7)
              n153 = Bundle(cluster=T5 {"Name"="", "Engine State"=enum."Initializing", "Engine Error"={"status"=FALSE, "code"=0, "source"=""}}, "Name"=w524, "Engine State"=w525, "Engine Error"=w526) -> (w528:T5)
            }
            n154 = call "send engine statuses.vi"("error in"=w521, "statuses"=w518, "message queue in"=w519) -> ("error out"=w520:errorcluster)  [unwired: 7 in, 1 out]
          }
        }
        n155 = feedback-in #1(w30) -> ()
      }
      frame True {
      }
    }
  }
  n156 = call <vilib>:"Destroy Message Queue.vi"("message queue in"=w2, "error in"=w14) -> ("error out"=w4:errorcluster)  [unwired: 11 in, 2 out]
  n157 = call <vilib>:"Destroy Message Queue.vi"("message queue in"=w1, "error in"=w4) -> ("error out"=w3:errorcluster)  [unwired: 11 in, 2 out]
  "error out" <- w3
  n158 = disable-structure shown="RUN_TIME_ENGINE==True" {
    disable-tunnel: w3 -> [_ _]
    frame condition #0 (active) {
    }
    frame condition #1 {
      n159 = call <vilib>:"Restart.vi"("Session in"=refnum<k21> "localhost" ("session in")) -> ()  [unwired: 8 in, 3 out]
    }
  }
